vi "KymeraPan.vi"(8 "error in (no error)":errorcluster caption="entrée d'erreur (pas d'erreur)", 11 "AndorSpectro.lvclass":refnum<class "AndorSpectro.lvclass">) -> (0 "error out":errorcluster caption="sortie d'erreur", 3 "AndorSpectro.lvclass Out":refnum<class "AndorSpectro.lvclass">)   [LabVIEW 2019, in "AndorSpectro.lvclass"]
uses:
  AndorSpectro.lvclass
  C:/Programmes Labview/LabscanV1A/DevicesClass/BaseDevice/BaseDevice.lvclass
  BaseDevice/Accessor/GetClassEvent.vi
  <userlib>/ATSpectrograph/atspectrograph.lvlib
panel:
  out "blaze out":string
  out "offset out":i32
  out "lines out":sgl
  out "home out":i32
  out "noGratings out":i32
  out "ChangeRef":refnum<vi>
  in  "numberPixels":i32=1024
  in  "CamUpdate":bool
  out "CalValuesRef":refnum<vi>
  out "WavelenghtRef":refnum<vi>
  out "CalValues":sgl[](array[numeric])
  in  "X Start":i32=1 min=1 max=1023 step=1
  in  "X End":i32=1024 min=2 max=1024 step=1
  in  "Graph Number":i32 min=0 max=256 step=1
  in  "AndorTabs":enum32{"Main Controls", "Settings"}(tab)
  out "Top Wl":sgl=100.0 caption="Top Wl. (nm)" min=0 max=3000 step=0.01
  out "Bot Wl":sgl=100.0 caption="Bot Wl. (nm)" min=0 max=3000 step=0.01
  in  "Output Port":i32(ring) caption="Device Name" items=["Direct", "Side"]
  in  "Input Port":i32(ring) caption="Device Name" items=["Direct", "Side"]
  in  "Con/Disc.":bool
  in  "Grating":i32(ring)=1 caption="Device Name" items=["G1 600L Blz 650"=1, "G2 1200L Blz 600"=2]
  in  "Wavelenght":sgl=100.0 caption="Center Wl. (nm)" min=0 max=3000 step=0.01
  in  "Focus (steps)":u16=1 min=1 max=500 step=1
  out "Moving":bool
  out "Grating offset":i32
  out "Detector offset":i32
  in  "MainProgQ":refnum<queue>
  in  "MainProgQEvent":refnum<user-event>
  in  "Acq":bool
  in  "Stop":bool
  out "Init Program":bool
  # "Andor Spectro"
  # "this MUST labeled with class name"
  # "this MUST be present and labeled \"Stop\" and \"Acq\""
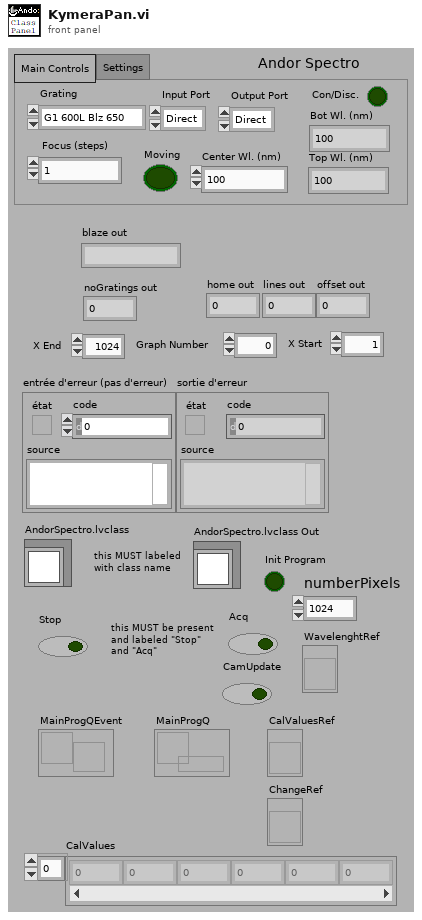
[diagram p1: front panel]
types:
  T1 = cluster{"Message":string, "Data":variant, "Code":i32}
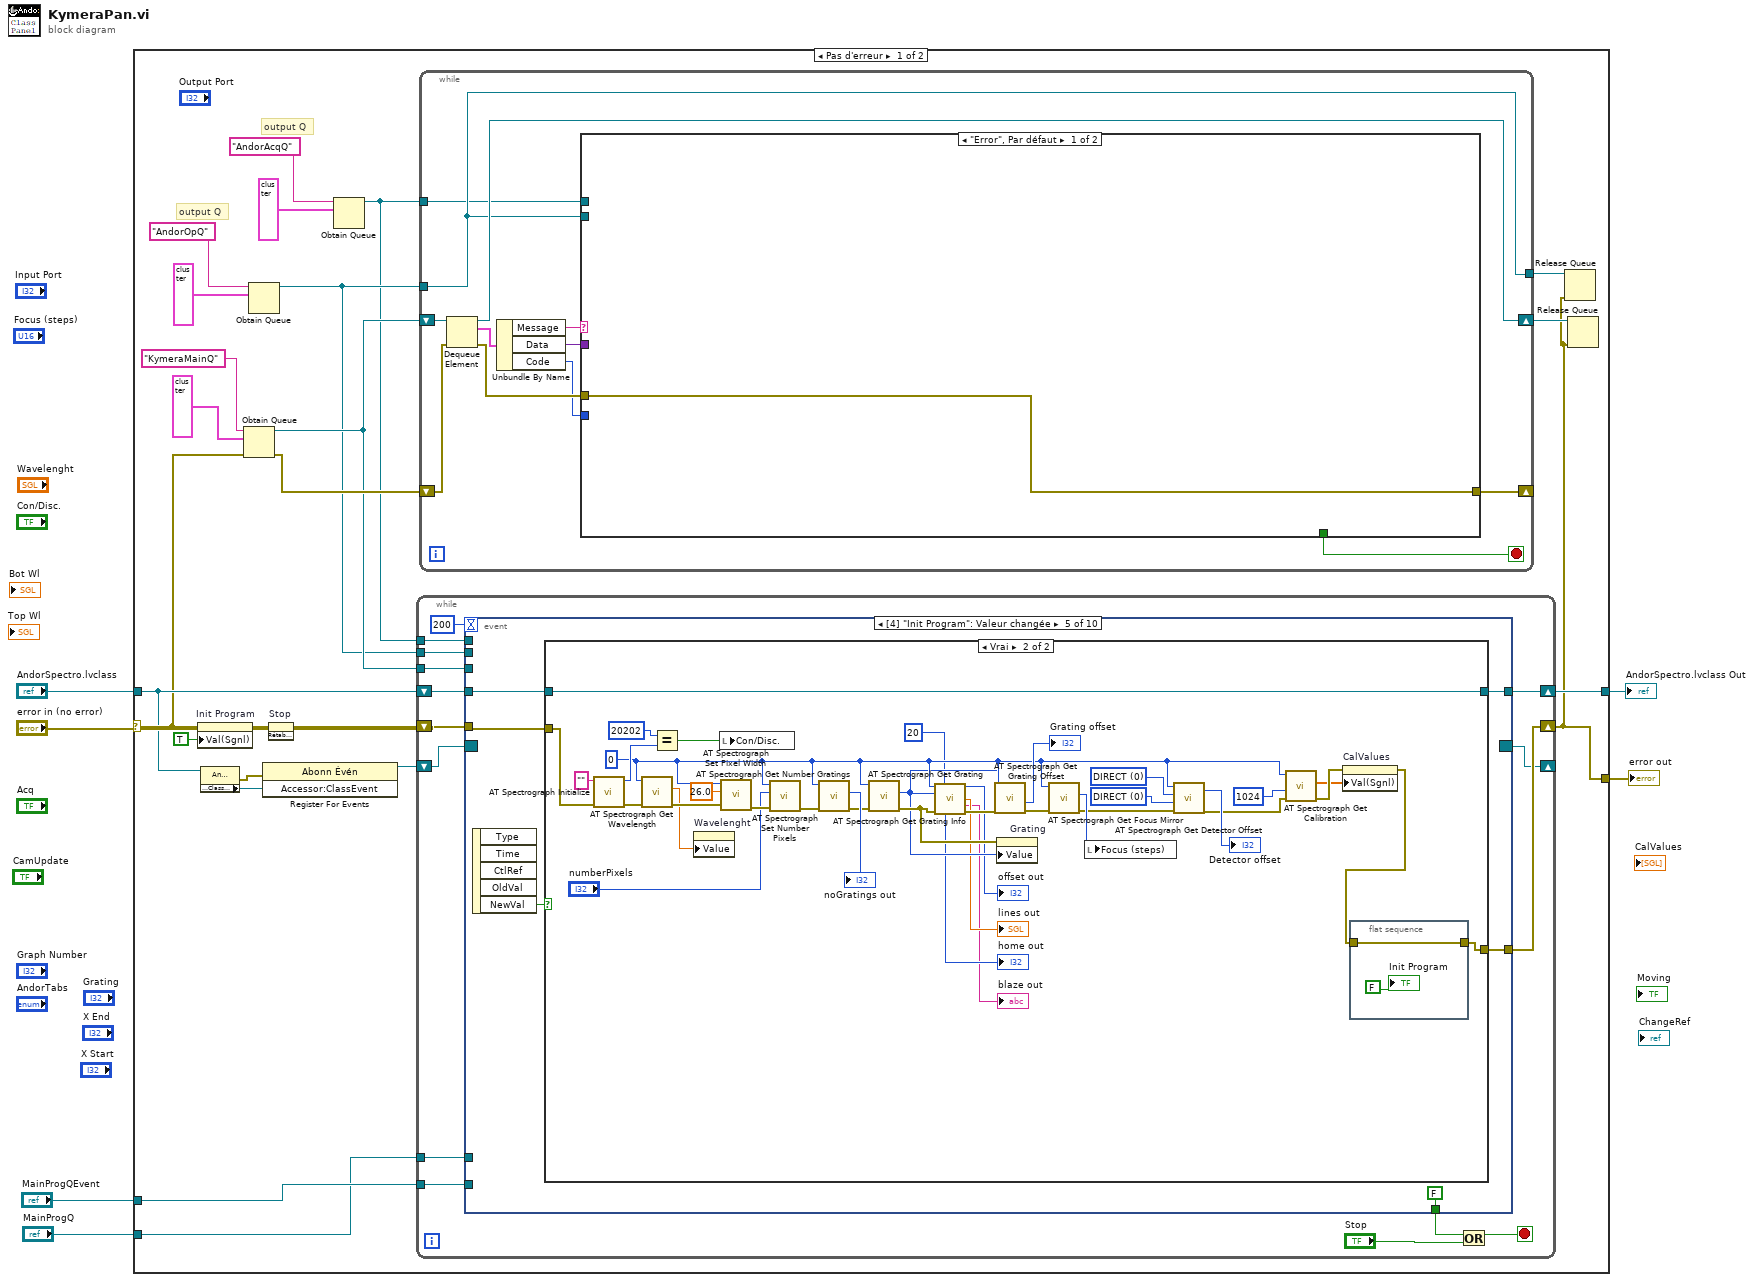
[diagram p0: block diagram]
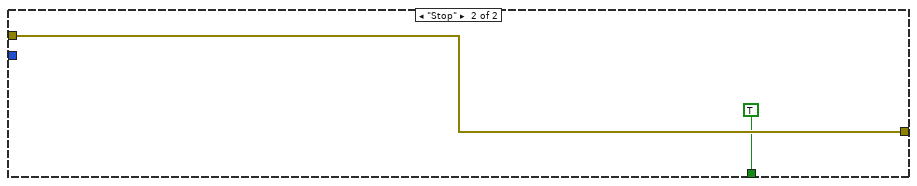
[diagram p2: hidden frame]
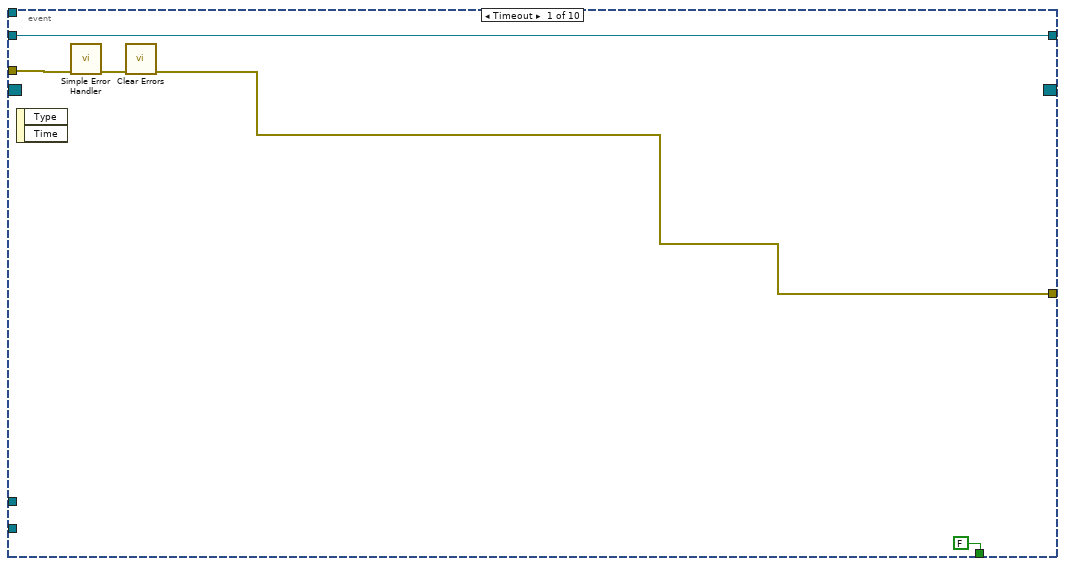
[diagram p3: hidden frame]
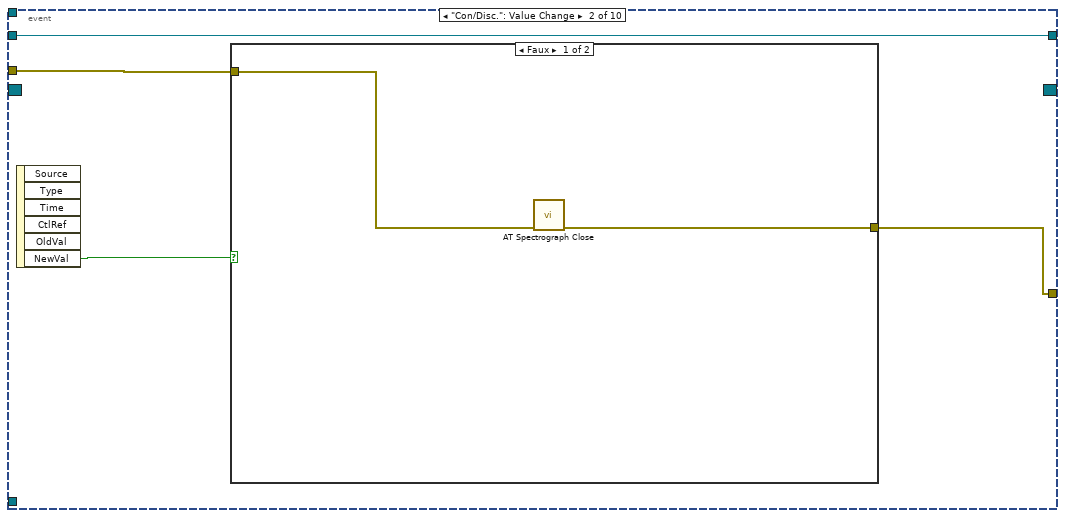
[diagram p4: hidden frame]
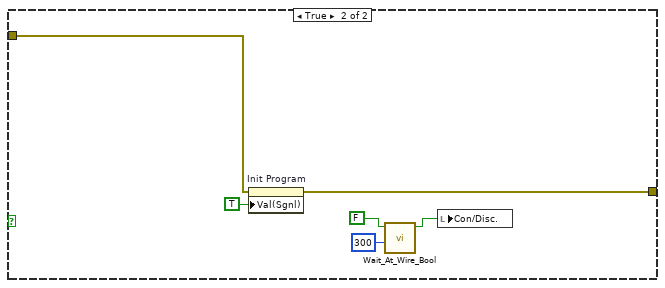
[diagram p5: hidden frame]
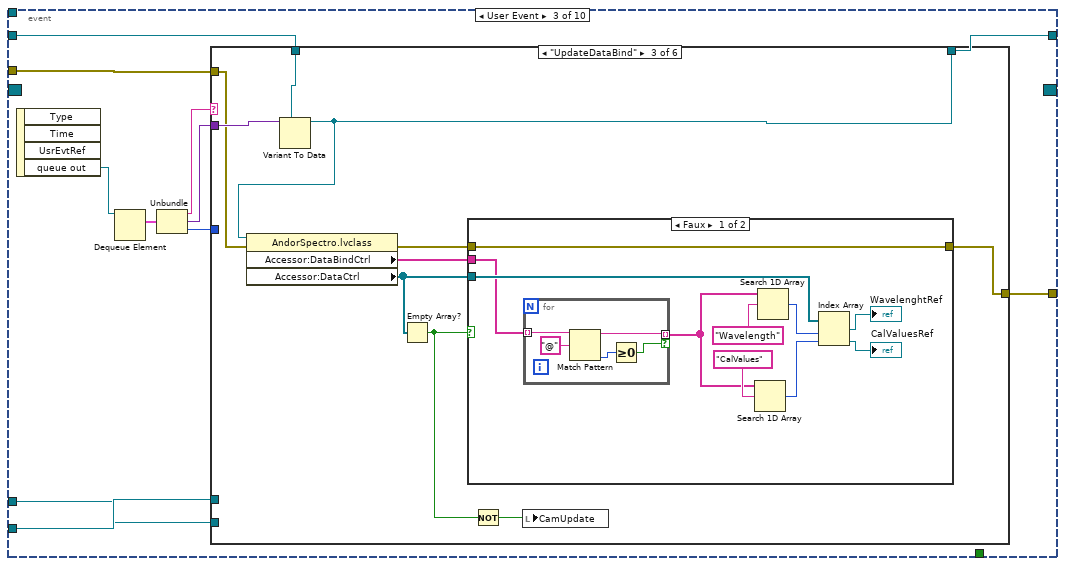
[diagram p6: hidden frame]
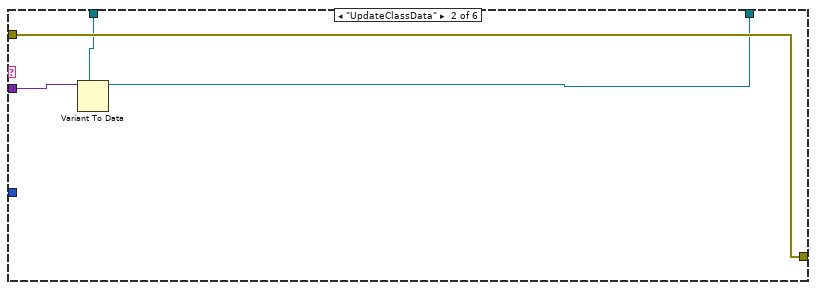
[diagram p8: hidden frame]
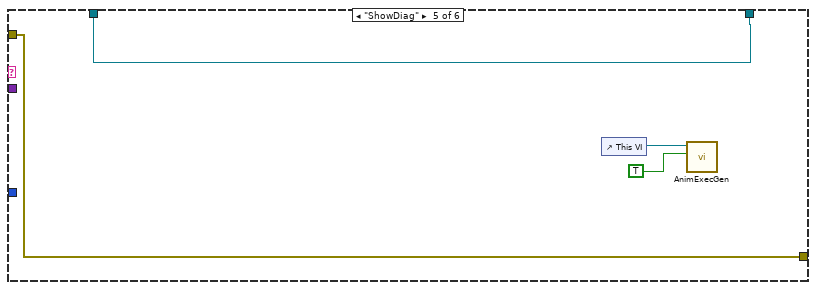
[diagram p11: hidden frame]
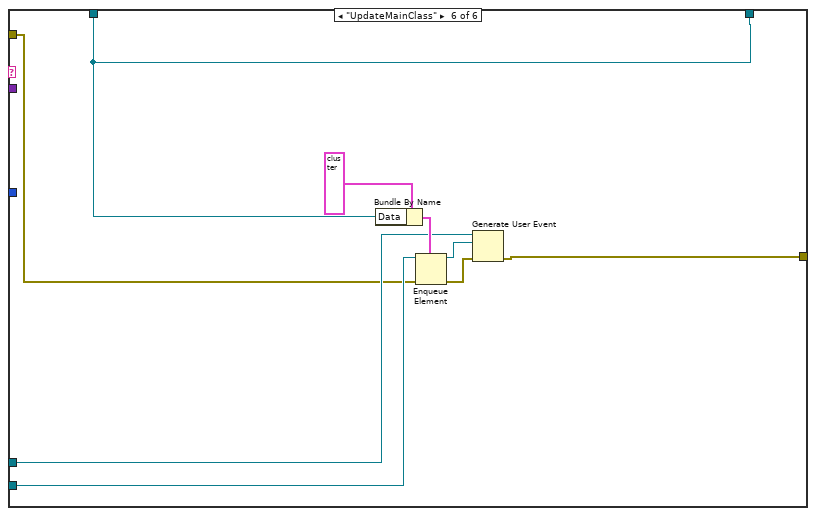
[diagram p12: hidden frame]
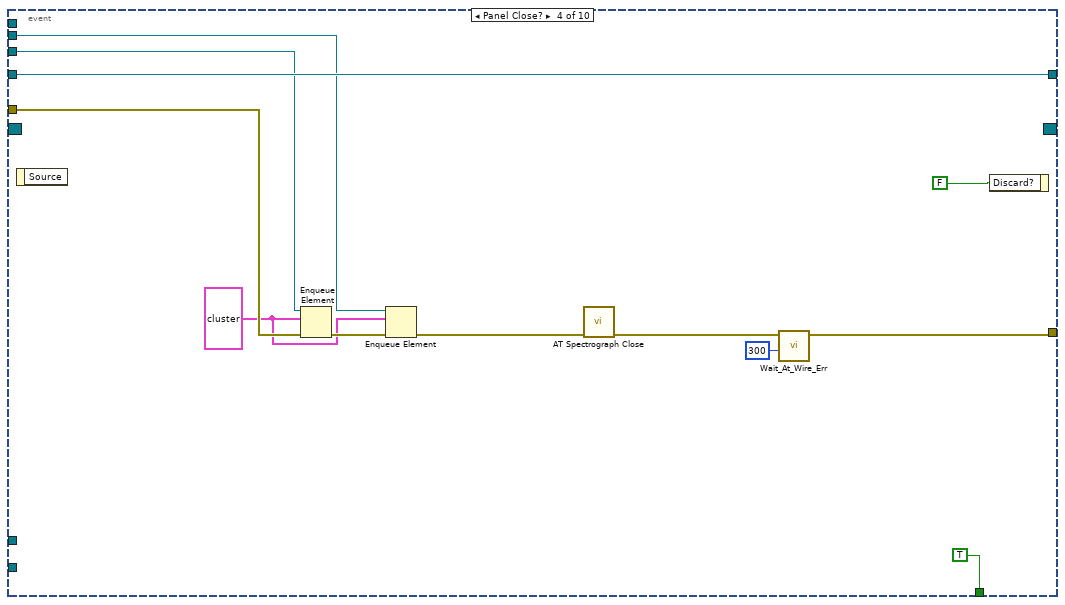
[diagram p13: hidden frame]
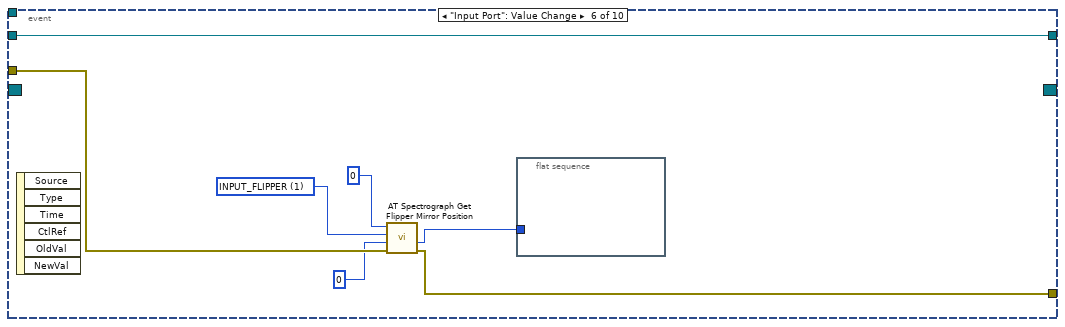
[diagram p15: hidden frame]
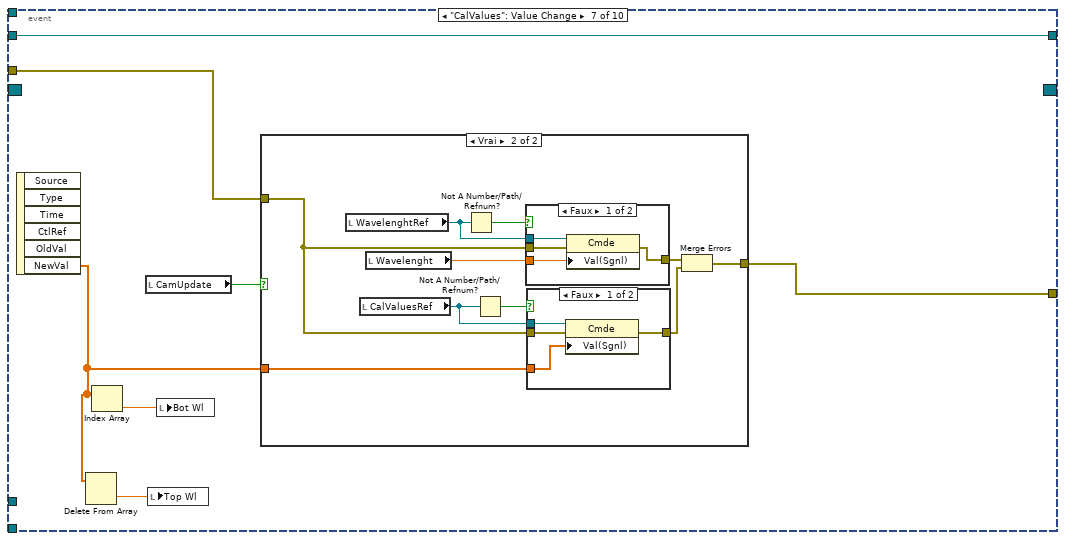
[diagram p16: hidden frame]
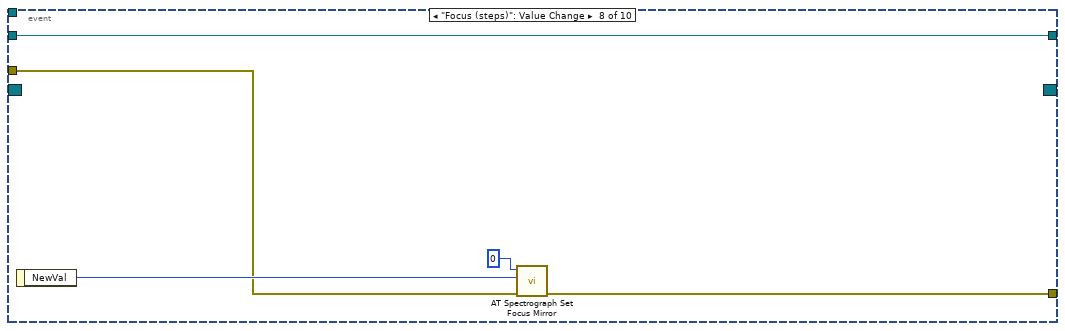
[diagram p20: hidden frame]
diagram:
  n1 = case shown="Pas d'erreur" "error in (no error)" {
    selector: "error in (no error)" -> [w20 w270]
    tunnel: [w8 w270] -> w5
    tunnel: "AndorSpectro.lvclass" -> [w25 w269]
    tunnel: [w29 w269] -> w3
    tunnel: "MainProgQEvent" -> [w23 _]
    tunnel: "MainProgQ" -> [w22 _]
    frame No Error {
      # "output Q"
      # "output Q"
      n2 = property on="Init Program" class="Bool (strict)"(error in=w20, "Val(Sgnl)"=TRUE ("Valeur (Signalisation)")) -> (error out=w28:errorcluster)  [unwired: 1 in, 1 out]
      n3 = property class="AndorSpectro.lvclass"(reference=w25) -> (error out=w27:errorcluster, "Accessor:ClassEvent"=w26:refnum<user-event>)  [unwired: 1 in, 1 out]
      n4 = Obtain Queue(name (unnamed)="KymeraMainQ" ("nom (aucun)"), element data type=T1 {"Message"="", "Data"=variant, "Code"=0}, error in (no error)=w20) -> (queue out=w17:refnum<queue>, error out=w19:errorcluster)  [unwired: 2 in, 1 out]
      n5 = Obtain Queue(name (unnamed)="AndorOpQ" ("nom (aucun)"), element data type=T1 {"Message"="", "Data"=variant, "Code"=0} ("element")) -> (queue out=w12:refnum<queue>)  [unwired: 3 in, 2 out]
      n6 = register-events(error in=w27, w26) -> (reference out=w24:refnum<event-registration>)  [unwired: 1 in, 1 out]
      n7 = invoke on="Stop" class="Bool (strict)" method="RétablirValParDéfaut"(error in=w28) -> (error out=w7:errorcluster)  [unwired: 2 in, 2 out]
      n8 = Obtain Queue(name (unnamed)="AndorAcqQ" ("nom (aucun)"), element data type=T1 {"Message"="", "Data"=variant, "Code"=0} ("element")) -> (queue out=w9:refnum<queue>)  [unwired: 3 in, 2 out]
      n9 = while {
        shift-right: [w58] -> w8
        shift-left: w7 -> [w59]
        shift-right: [w55] -> w29
        shift-left: w25 -> [w57]
        shift-right: [w51] -> _
        shift-left: w24 -> [w52]
        tunnel: w23 -> [w50]
        tunnel: w22 -> [w49]
        tunnel: w17 -> [w48]
        tunnel: w12 -> [w47]
        tunnel: w9 -> [w46]
        stop <- w54 stop-if-true
        n10 = event shown="[4] \"Init Program\": Valeur changée" {
          selector: w52 -> [_ _ _ _ _ _ _ _ _ _]
          dyn-events: [_ _ _ _ _ _ _ _ _ _] -> w51
          timeout: 200 -> [_ _ _ _ _ _ _ _ _ _]
          tunnel: w59 -> [w63 w68 w87 w143 w150 w200 w206 w232 w244 w267]
          tunnel: [w61 w66 w81 w138 w152 w199 w205 w231 w242 w255] -> w58
          tunnel: w57 -> [w64 w67 w88 w145 w149 w201 w208 w233 w245 w268]
          tunnel: [FALSE _ _ TRUE FALSE _ _ _ _ _] -> w56
          tunnel: [w64 w67 w80 w145 w148 w201 w208 w233 w245 w268] -> w55
          tunnel: w50 -> [_ _ w79 _ _ _ _ _ _ _]
          tunnel: w49 -> [_ _ w78 _ _ _ _ _ _ _]
          tunnel: w48 -> [_ _ _ w144 _ _ _ _ _ _]
          tunnel: w47 -> [_ _ _ w140 _ _ _ _ _ _]
          tunnel: w46 -> [_ _ _ _ _ _ _ _ _ _]
          event Timeout {
            n11 = event-data() -> ()  [unwired: 1 in, 2 out]
            n12 = call <vilib>:"Simple Error Handler.vi"("error in (no error)"=w63) -> ("error out"=w62:errorcluster)  [unwired: 4 in, 4 out]
            n13 = call <vilib>:"Clear Errors.vi"("error in (no error)"=w62) -> ("error out"=w61:errorcluster)  [unwired: 5 in, 1 out]
          }
          event "Con/Disc.": Value Change {
            n14 = event-data() -> ("NewVal"=w69:bool)  [unwired: 1 in, 5 out]
            n15 = case shown="Faux" w69 {
              tunnel: w68 -> [w70 w76]
              tunnel: [w71 w75] -> w66
              frame False {
                n16 = call <userlib>:"AT Spectrograph Close.vi"("error in (no error)"=w70) -> ("error out"=w71:errorcluster)  [unwired: 9 in, 1 out]
              }
              frame True {
                n17 = property on="Init Program" class="Bool (strict)"(error in=w76, "Val(Sgnl)"=TRUE ("Valeur (Signalisation)")) -> (error out=w75:errorcluster)  [unwired: 1 in, 1 out]
                n18 = call <userlib>:"Wait_At_Wire_Bool.vi"("Wait (ms)"=u32 300, "error in (no error)"=FALSE ("Con/Disc.")) -> ("error out"=w73:bool)  [unwired: 7 in, 2 out]
                n19 = local write "Con/Disc."(w73) -> ()
              }
            }
          }
          event User Event {
            n20 = event-data() -> ("queue out"=w85:refnum<queue>)  [unwired: 1 in, 3 out]
            n21 = Dequeue Element(queue=w85) -> (element=w86:cluster{"Message":string, "Data":variant, i32})  [unwired: 2 in, 3 out]
            n22 = Unbundle(w86) -> ("Message"=w84:string, "Data"=w83:variant, w82:i32)
            n23 = case shown="\"UpdateDataBind\"" w84 {
              tunnel: w87 -> [w90 w94 w96 w121 w125 w128]
              tunnel: w83 -> [_ w93 w104 _ _ _]
              tunnel: w88 -> [w89 w92 w103 w122 w126 w131]
              tunnel: [w89 w91 w97 w122 w126 w131] -> w80
              tunnel: [w90 w94 w95 w121 w125 w127] -> w81
              tunnel: w82 -> [_ _ _ _ _ _]
              tunnel: w79 -> [_ _ _ _ _ w130]
              tunnel: w78 -> [_ _ _ _ _ w129]
              frame Default {
              }
              frame "UpdateClassData" {
                n24 = Variant To Data(type=w92, Variant=w93) -> (data=w91:refnum<class "AndorSpectro.lvclass">)  [unwired: 1 in, 1 out]
              }
              frame "UpdateDataBind" {
                n25 = Variant To Data(type=w103, Variant=w104) -> (data=w97:refnum<class "AndorSpectro.lvclass">)  [unwired: 1 in, 1 out]
                n26 = property class="AndorSpectro.lvclass"(reference=w97, error in=w96) -> (error out=w100:errorcluster, "Accessor:DataBindCtrl"=w102:string[], "Accessor:DataCtrl"=w101:refnum<vi>[])  [unwired: 1 out]
                n27 = Empty Array?(array=w101) -> (empty?=w99:bool)
                n28 = case shown="Faux" w99 {
                  tunnel: w102 -> [w106 _]
                  tunnel: w101 -> [w110 _]
                  tunnel: w100 -> [w107 w120]
                  tunnel: [w107 w120] -> w95
                  frame False {
                    n29 = for {
                      tunnel: w106 -> [w119] mode=indexing
                      tunnel: [w117] -> w105 mode=indexing if=w116
                      n30 = Match Pattern(string=w119, regular expression="@" ("expression régulière")) -> (before substring=w117:string, offset past match=w115:i32)  [unwired: 1 in, 2 out]
                      n31 = Greater Or Equal To 0?(x=w115) -> (x >= 0?=w116:bool)
                    }
                    n32 = Search 1D Array(1D array=w105, element="CalValues" ("nom (aucun)")) -> (index of element=w111:i32)  [unwired: 1 in]
                    n33 = Search 1D Array(1D array=w105, element="Wavelength" ("nom (aucun)")) -> (index of element=w113:i32)  [unwired: 1 in]
                    n34 = Index Array(array=w110, index #1=w113, index #2=w111) -> (element #1=→"WavelenghtRef":refnum<vi>, element #2=→"CalValuesRef":refnum<vi>)
                  }
                  frame True {
                  }
                }
                n35 = Not(x=w99) -> (.not. x?=w98:bool)
                n36 = local write "CamUpdate"(w98) -> ()
              }
              frame "MeasDone" {
              }
              frame "ShowDiag" {
                n37 = control-ref of="This VI"() -> (w124:refnum<vi>)
                n38 = call <userlib>:"AnimExecGen.vi"("Animer l'exécution ?"=TRUE, "ViRef"=w124) -> ()  [unwired: 9 in, 1 out]
              }
              frame "UpdateMainClass" {
                n39 = Bundle By Name(cluster=cluster{"Message":string, "Data":variant, i32} {"Message"="", "Data"=variant, 0} ("élément"), "Data"=w131) -> (w132:cluster{"Message":string, "Data":variant, i32})
                n40 = Enqueue Element(queue=w129, element=w132, error in (no error)=w128) -> (queue out=w135:refnum<queue>, error out=w134:errorcluster)  [unwired: 1 in, 1 out]
                n41 = Generate User Event(user event=w130, event data cluster=w135, error in=w134) -> (error out=w127:errorcluster)  [unwired: 1 in, 1 out]
              }
            }
          }
          event Panel Close? {
            w139 = T1 {"Message"="Stop", "Data"=variant, "Code"=0} ("élément")
            n42 = event-data() -> ()  [unwired: 1 in, 1 out]
            n43 = Enqueue Element(queue=w144, element=w139, error in (no error)=w143) -> (error out=w141:errorcluster)  [unwired: 1 in, 2 out]
            n44 = Enqueue Element(queue=w140, element=w139, error in (no error)=w141) -> (error out=w136:errorcluster)  [unwired: 1 in, 2 out]
            n45 = call <userlib>:"AT Spectrograph Close.vi"("error in (no error)"=w136) -> ("error out"=w142:errorcluster)  [unwired: 9 in, 1 out]
            n46 = call <userlib>:"Wait_At_Wire_Err.vi"("Wait (ms)"=u32 300, "error in (no error)"=w142) -> ("error out"=w138:errorcluster)  [unwired: 7 in, 2 out]
            n47 = event-data("Discard?"=FALSE ("Rejeter ?")) -> ()  [unwired: 1 in, 1 out]
          }
          event "Init Program": Value Change {
            n48 = event-data() -> ("NewVal"=w153:bool)  [unwired: 1 in, 4 out]
            n49 = case shown="Vrai" w153 {
              tunnel: w150 -> [w155 w177]
              tunnel: [w155 w176] -> w152
              tunnel: w149 -> [w154 w175]
              tunnel: [w154 w175] -> w148
              frame False {
              }
              frame True {
                w186 = u32 0 items=["DIRECT", "SIDE"] ("entrancePort")
                w187 = u32 0 items=["DIRECT", "SIDE"] ("exitPort")
                w163 = 0
                n50 = call <userlib>:"AT Spectrograph Initialize.vi"("error in (no error)"=w177, "iniPath"="") -> ("error out"=w183:errorcluster, "function return"=w179:u32)  [unwired: 8 in]
                n51 = call <userlib>:"AT Spectrograph Get Wavelength.vi"("error in (no error)"=w183, "device"=w163) -> ("error out"=w182:errorcluster, "wavelength out"=w174:sgl)  [unwired: 7 in, 1 out]
                n52 = Equal?(x=u32 20202, y=w179) -> (x = y?=w178:bool)
                n53 = property on="Wavelenght" class="NumNb (strict)"("Value"=w174) -> ()  [unwired: 2 in, 2 out]
                n54 = local write "Con/Disc."(w178) -> ()
                n55 = call <userlib>:"AT Spectrograph Set Pixel Width.vi"("error in (no error)"=w182, "width"=sgl 26.0, "device"=w163) -> ("error out"=w190:errorcluster)  [unwired: 7 in, 1 out]
                n56 = call <userlib>:"AT Spectrograph Set Number Pixels.vi"("error in (no error)"=w190, "numberPixels"="numberPixels", "device"=w163) -> ("error out"=w167:errorcluster)  [unwired: 7 in, 1 out]
                n57 = call <userlib>:"AT Spectrograph Get Number Gratings.vi"("error in (no error)"=w167, "device"=w163) -> ("error out"=w157:errorcluster, "noGratings out"=→"noGratings out":i32)  [unwired: 7 in, 1 out]
                n58 = call <userlib>:"AT Spectrograph Get Grating.vi"("error in (no error)"=w157, "device"=w163) -> ("error out"=w164:errorcluster, "grating out"=w162:i32)  [unwired: 7 in, 1 out]
                n59 = call <userlib>:"AT Spectrograph Get Grating Info.vi"("device"=w163, "maxBlazeStrLen"=20, "grating"=w162, "error in (no error)"=w164) -> ("offset out"=→"offset out":i32, "lines out"=→"lines out":sgl, "blaze out"=→"blaze out":string, "home out"=→"home out":i32, "error out"=w165:errorcluster)  [unwired: 6 in, 1 out]
                n60 = call <userlib>:"AT Spectrograph Get Grating Offset.vi"("error in (no error)"=w165, "grating"=w162, "device"=w163) -> ("error out"=w171:errorcluster, "offset out"=→"Grating offset":i32)  [unwired: 6 in, 1 out]
                n61 = property on="Grating" class="MDér (strict)"(error in=w164, "Value"=w162) -> ()  [unwired: 1 in, 2 out]
                n62 = call <userlib>:"AT Spectrograph Get Focus Mirror.vi"("error in (no error)"=w171, "device"=w163) -> ("error out"=w169:errorcluster, "focus out"=w170:i32)  [unwired: 7 in, 1 out]
                n63 = local write "Focus (steps)"(w170) -> ()
                n64 = call <userlib>:"AT Spectrograph Get Detector Offset.vi"("error in (no error)"=w169, "exitPort"=w187, "entrancePort"=w186, "device"=w163) -> ("error out"=w180:errorcluster, "offset out"=→"Detector offset":i32)  [unwired: 5 in, 1 out]
                n65 = call <userlib>:"AT Spectrograph Get Calibration.vi"("error in (no error)"=w180, "numberPixels"=1024, "device"=w163) -> ("error out"=w173:errorcluster, "calibrationValuesOut"=w172:sgl[])  [unwired: 5 in, 1 out]
                n66 = property on="CalValues" class="Tabl (strict)"(error in=w173, "Val(Sgnl)"=w172) -> (error out=w168:errorcluster)  [unwired: 1 in, 1 out]
                n67 = flat-sequence {
                  tunnel: [w193] -> w176
                  tunnel: w168 -> [w193]
                  frame #0 {
                    "Init Program" <- FALSE
                  }
                }
              }
            }
          }
          event "Input Port": Value Change {
            w197 = u32 1 items=["INPUT_FLIPPER"=1, "OUTPUT_FLIPPER"=2] ("flipper")
            n68 = event-data() -> ()  [unwired: 1 in, 6 out]
            n69 = call <userlib>:"AT Spectrograph Get Flipper Mirror Position.vi"("error in (no error)"=w200, "position"=0, "flipper"=w197, "device"=0) -> ("error out"=w199:errorcluster, "position out"=w195:i32)  [unwired: 5 in, 1 out]
            n70 = flat-sequence {
              tunnel: w195 -> [_]
              frame #0 {
              }
            }
          }
          event "CalValues": Value Change {
            n71 = event-data() -> ("NewVal"=w203:sgl[])  [unwired: 1 in, 5 out]
            n72 = Delete From Array(array=w203) -> (deleted portion=w202:sgl)  [unwired: 2 in, 1 out]
            n73 = Index Array(array=w203) -> (element=w204:sgl)  [unwired: 1 in]
            n74 = local read "CamUpdate"() -> (w207:bool)
            n75 = local write "Top Wl"(w202) -> ()
            n76 = local write "Bot Wl"(w204) -> ()
            n77 = case shown="Vrai" w207 {
              tunnel: w206 -> [w209 w215]
              tunnel: w203 -> [_ w214]
              tunnel: [w209 w210] -> w205
              frame False {
              }
              frame True {
                n78 = local read "WavelenghtRef"() -> (w211:refnum<vi>)
                n79 = local read "CalValuesRef"() -> (w213:refnum<vi>)
                n80 = local read "Wavelenght"() -> (w212:sgl)
                n81 = Not A Number/Path/Refnum?(number/path/refnum=w211) -> (NaN/Path/Refnum?=w216:bool)
                n82 = Not A Number/Path/Refnum?(number/path/refnum=w213) -> (NaN/Path/Refnum?=w217:bool)
                n83 = case shown="Faux" w216 {
                  tunnel: w211 -> [w228 _]
                  tunnel: w212 -> [w227 _]
                  tunnel: w215 -> [w226 w229]
                  tunnel: [w225 w229] -> w218
                  frame False {
                    n84 = property class="Cmde"(reference=w228, error in=w226, "Val(Sgnl)"=w227) -> (error out=w225:errorcluster)  [unwired: 1 out]
                  }
                  frame True {
                  }
                }
                n85 = case shown="Faux" w217 {
                  tunnel: w213 -> [w223 _]
                  tunnel: w215 -> [w220 w224]
                  tunnel: [w222 w224] -> w219
                  tunnel: w214 -> [w221 _]
                  frame False {
                    n86 = property class="Cmde"(reference=w223, error in=w220, "Val(Sgnl)"=w221) -> (error out=w222:errorcluster)  [unwired: 1 out]
                  }
                  frame True {
                  }
                }
                n87 = Merge Errors(w218, w219) -> (w210:errorcluster)
              }
            }
          }
          event "Focus (steps)": Value Change {
            n88 = event-data() -> ("NewVal"=w234:u16)  [unwired: 1 in]
            n89 = call <userlib>:"AT Spectrograph Set Focus Mirror.vi"("error in (no error)"=w232, "focus"=w234, "device"=0) -> ("error out"=w231:errorcluster)  [unwired: 7 in, 1 out]
          }
          event "Wavelenght": Value Change {
            w238 = 0 ("device")
            n90 = event-data() -> ("NewVal"=w243:sgl)  [unwired: 1 in, 5 out]
            n91 = call <userlib>:"AT Spectrograph Set Wavelength.vi"("error in (no error)"=w244, "wavelength"=w243, "device"=w238) -> ("error out"=w237:errorcluster)  [unwired: 7 in, 1 out]
            n92 = call <userlib>:"AT Spectrograph Get Wavelength.vi"("error in (no error)"=w237, "device"=w238) -> ("error out"=w236:errorcluster, "wavelength out"=w235:sgl)  [unwired: 7 in, 1 out]
            n93 = local write "Wavelenght"(w235) -> ()
            n94 = call <userlib>:"AT Spectrograph Get Calibration.vi"("error in (no error)"=w236, "numberPixels"=1024, "device"=w238) -> ("error out"=w240:errorcluster, "calibrationValuesOut"=w239:sgl[])  [unwired: 5 in, 1 out]
            n95 = property on="CalValues" class="Tabl (strict)"(error in=w240, "Val(Sgnl)"=w239) -> (error out=w242:errorcluster)  [unwired: 1 in, 1 out]
          }
          event "Grating": Value Change {
            w254 = 0 ("device")
            n96 = event-data() -> ("NewVal"=w266:i32)  [unwired: 1 in]
            n97 = local read "Grating"() -> (w257:i32)
            n98 = call <userlib>:"AT Spectrograph Set Grating.vi"("error in (no error)"=w267, "grating"=w266, "device"=w254) -> ("error out"=w259:errorcluster)  [unwired: 7 in, 1 out]
            n99 = call <userlib>:"AT Spectrograph Get Grating.vi"("error in (no error)"=w259, "grating"=w257) -> ("error out"=w258:errorcluster, "grating out"=w253:i32)  [unwired: 7 in, 1 out]
            n100 = local write "Grating"(w253) -> ()
            n101 = call <userlib>:"AT Spectrograph Get Focus Mirror.vi"("error in (no error)"=w258, "device"=w254) -> ("error out"=w263:errorcluster, "focus out"=w262:i32)  [unwired: 7 in, 1 out]
            n102 = call <userlib>:"AT Spectrograph Get Wavelength.vi"("error in (no error)"=w263, "device"=w254) -> ("error out"=w252:errorcluster, "wavelength out"=w264:sgl)  [unwired: 7 in, 1 out]
            n103 = local write "Focus (steps)"(w262) -> ()
            n104 = property on="Wavelenght" class="NumNb (strict)"(error in=w252, "Value"=w264) -> (error out=w251:errorcluster)  [unwired: 1 in, 1 out]
            n105 = call <userlib>:"AT Spectrograph Get Calibration.vi"("error in (no error)"=w251, "numberPixels"=1024, "device"=w254) -> ("error out"=w261:errorcluster, "calibrationValuesOut"=w260:sgl[])  [unwired: 5 in, 1 out]
            n106 = property on="CalValues" class="Tabl (strict)"(error in=w261, "Val(Sgnl)"=w260) -> (error out=w256:errorcluster)  [unwired: 1 in, 1 out]
            n107 = call <userlib>:"AT Spectrograph Get Grating Info.vi"("device"=w254, "maxBlazeStrLen"=20, "grating"=w253, "error in (no error)"=w256) -> ("offset out"=w247:i32, "lines out"=w249:sgl, "blaze out"=w250:string, "home out"=w248:i32, "error out"=w255:errorcluster)  [unwired: 6 in, 1 out]
            n108 = local write "blaze out"(w250) -> ()
            n109 = local write "home out"(w248) -> ()
            n110 = local write "lines out"(w249) -> ()
            n111 = local write "offset out"(w247) -> ()
          }
        }
        n112 = Or(x=w56, y="Stop") -> (x .or. y?=w54:bool)
      }
      n113 = while {
        shift-right: [w41] -> w14
        shift-left: w17 -> [w42]
        shift-right: [w38] -> _
        shift-left: w19 -> [w36]
        tunnel: w12 -> [w33]
        tunnel: [w33] -> w13
        tunnel: w9 -> [w32]
        stop <- w35 stop-if-true
        n114 = Dequeue Element(queue=w42, error in (no error)=w36) -> (queue out=w41:refnum<queue>, element=w40:T1, error out=w37:errorcluster)  [unwired: 1 in, 1 out]
        n115 = Unbundle By Name(w40) -> ("Message"=w39:string, "Data"=w34:variant, "Code"=w31:i32)
        n116 = case shown="\"Error\", Par défaut" w39 {
          tunnel: [w43 w45] -> w38
          tunnel: w37 -> [w43 w45]
          tunnel: [_ TRUE] -> w35
          tunnel: w34 -> [_ _]
          tunnel: w33 -> [_ _]
          tunnel: w32 -> [_ _]
          tunnel: w31 -> [_ _]
          frame "Error", Default {
          }
          frame "Stop" {
          }
        }
      }
      n117 = Release Queue(queue=w13, error in (no error)=w8) -> ()  [unwired: 1 in, 3 out]
      n118 = Release Queue(queue=w14, error in (no error)=w8) -> ()  [unwired: 1 in, 3 out]
    }
    frame Error {
    }
  }
  "error out" <- w5
  "AndorSpectro.lvclass Out" <- w3
